vi "Close Instrument.vi"(8 "error in (no error)":errorcluster, 11 "Fluke DMM.lvclass in":refnum<class "Fluke DMM.lvclass">) -> (0 "error out":errorcluster, 3 "Fluke DMM.lvclass out":refnum<class "Fluke DMM.lvclass">)   [LabVIEW 2010, in "Fluke DMM.lvclass"]
uses:
  Fluke DMM.lvclass
  Fluke DMM.lvclass/Fluke DMM.ctl
  <instrlib>/Fluke 884X Series/Fluke 884X Series.lvlib
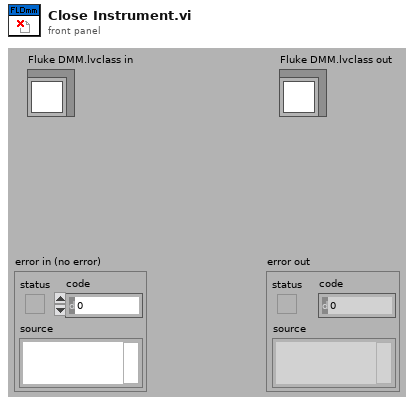
[diagram p1: front panel]
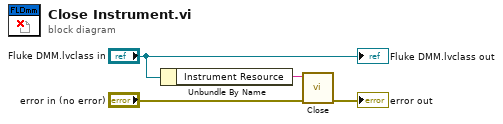
[diagram p0: block diagram]
diagram:
  n1 = Unbundle By Name("Fluke DMM.lvclass in") -> ("Instrument Resource"=w1:string)
  n2 = call <instrlib>:"Close.vi"("error in (no error)"="error in (no error)", "VISA resource name"=w1) -> ("error out"=→"error out":errorcluster)  [unwired: 9 out]
  "Fluke DMM.lvclass out" <- "Fluke DMM.lvclass in"
